vi "EMC_Coordinate_Move.vi"(6 "position[]":dbl[](array[numeric]), 7 "line move mode":i32(ring)=10551344 items=["Relative"=10551344, "Absolute"=10551337, "Relative To Capture"=10551345, "Velocity"=10551346, "Polyline"=11600101], 8 "error in (no error)":errorcluster, 9 "velocity":dbl=1000.0, 10 "Motion Parameters":T1={"position"=1000.0, "velocity"=1000.0, "acceleration"=10000.0, "deceleration"=10000.0, "accel. jerk"=10000.0, "decel. jerk"=10000.0}, 11 "resource":refnum<k21>) -> (0 "error out":errorcluster)   [LabVIEW 2015]
uses:
  EMC_Typedef_Motor_Parameters.ctl
  <vilib>/Motion/PropertyNodes/nimc.createStraightLineMoveInstance.coordinate.vi
  <vilib>/Motion/PropertyNodes/nimc.destroyInterfaceInstance.vi
  <resource>/objmgr/nimotion.rc
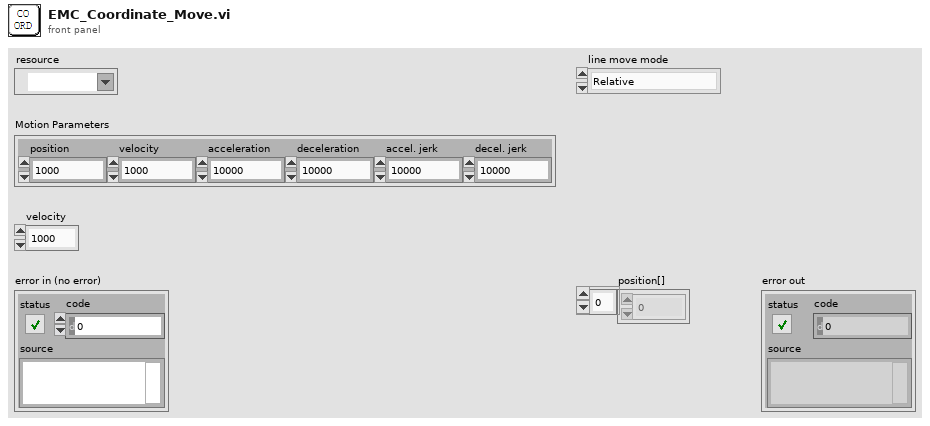
[diagram p1: front panel]
types:
  T1 = typedef "EMC_Typedef_Motor_Parameters.ctl" = cluster{"position":dbl, "velocity":dbl, "acceleration":dbl, "deceleration":dbl, "accel. jerk":dbl, "decel. jerk":dbl}
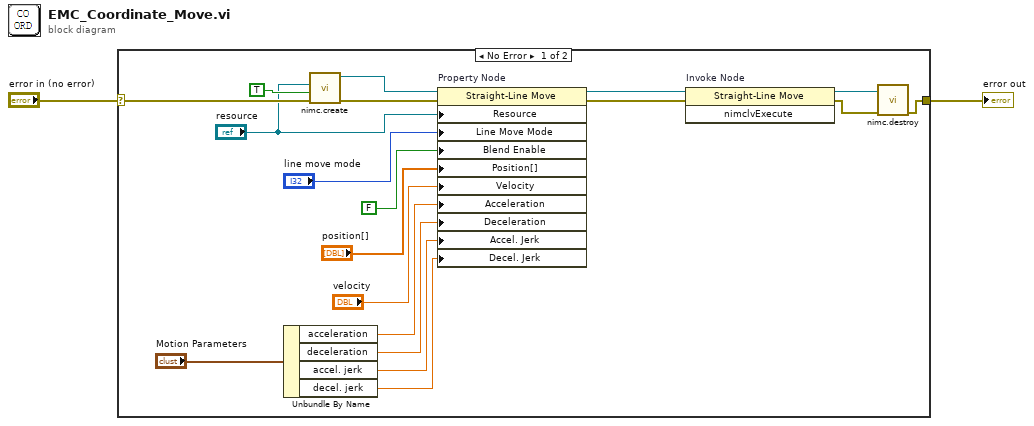
[diagram p0: block diagram]
diagram:
  n1 = case shown="No Error" "error in (no error)" {
    selector: "error in (no error)" -> [w20 w22]
    tunnel: [w3 w22] -> w1
    frame No Error {
      n2 = Unbundle By Name("Motion Parameters") -> ("acceleration"=w10:dbl, "deceleration"=w9:dbl, "accel. jerk"=w8:dbl, "decel. jerk"=w7:dbl)
      n3 = call-poly <vilib>:"nimc.create.vi"("error in"=w20, "async?"=TRUE, "coordinate"="resource") -> ("error out"=w6:errorcluster, "line"=w13:refnum<k20>)  [unwired: 6 in, 1 out]
      n4 = property on="Property Node" class="Straight-Line Move"(reference=w13, error in=w6, "Resource"="resource", "Line Move Mode"="line move mode", "Blend Enable"=FALSE ("blend enable"), "Position[]"="position[]", "Velocity"="velocity", "Acceleration"=w10, "Deceleration"=w9, "Accel. Jerk"=w8, "Decel. Jerk"=w7) -> (reference out=w18:refnum<k20>, error out=w19:errorcluster)
      n5 = invoke on="Invoke Node" class="Straight-Line Move" method="nimclvExecute"(reference=w18, error in=w19) -> (reference out=w5:refnum<k20>, error out=w4:errorcluster)  [unwired: 1 in, 1 out]
      n6 = call-poly <vilib>:"nimc.destroy.vi"("error in"=w4, "motion handle"=w5) -> ("error out"=w3:errorcluster)  [unwired: 9 in]
    }
    frame Error {
    }
  }
  "error out" <- w1
